vi "Array Manipulation.vi"() -> ()   [LabVIEW 2015]
panel:
  out "Sorted Array":dbl[](array[numeric])
  in  "Array Size":i32 format="%.0p"
  out "Sum":dbl format="%#.6p"
  out "Elements in Array":i32 format="%.1p"
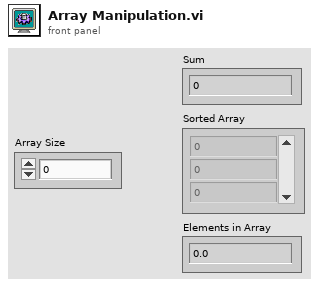
[diagram p1: front panel]
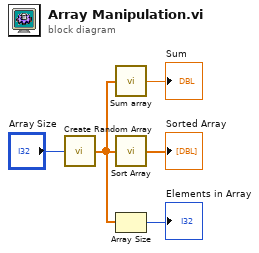
[diagram p0: block diagram]
diagram:
  n1 = call "Create Random Array.vi"("Array Size"="Array Size") -> ("Random Array Out"=w1:dbl[])
  n2 = call "Sum array.vi"("Array in"=w1) -> ("Sum"=→"Sum":dbl)
  n3 = call "Sort Array.vi"("Array In"=w1) -> ("Sorted Array Out"=→"Sorted Array":dbl[])
  n4 = Array Size(array=w1) -> (size(s)=→"Elements in Array":i32)
